vi "S_fi.vi"(6 "Parametry Ziemi":T1={"a - półoś duża"=6378137.0, "b - półoś mała"=6356752.3141999999998} {"b - półoś mała" format="%_20f"; "a - półoś duża" format="%_20g"}, 8 "E":ext, 9 "fi'":ext) -> (2 "S_fi":ext)   [LabVIEW 2015, in "Biblioteka moduł map v3.lvlib" / "Konwersja wsp.lvlib" / "UTM.lvlib" / "Konwersja z UTM na wsp geograficzne.lvlib"]
uses:
  Konwersja z UTM na wsp geograficzne.lvlib
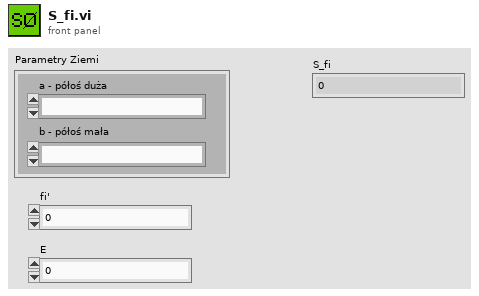
[diagram p1: front panel]
types:
  T1 = cluster{"a - półoś duża":ext, "b - półoś mała":ext}
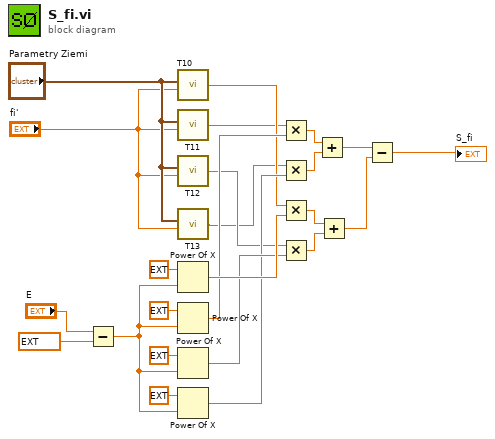
[diagram p0: block diagram]
diagram:
  n1 = Subtract(x="E", y=ext 500000.0 ("FE")) -> (x-y=w22:ext)
  n2 = call "T10.vi"("Parametry Ziemi"="Parametry Ziemi", "fi'"="fi'") -> ("T10"=w6:ext)  [unwired: 6 in]
  n3 = call "T11.vi"("Parametry Ziemi"="Parametry Ziemi", "fi'"="fi'") -> ("T11"=w5:ext)  [unwired: 6 in]
  n4 = call "T12.vi"("Parametry Ziemi"="Parametry Ziemi", "fi'"="fi'") -> ("T12"=w4:ext)  [unwired: 6 in]
  n5 = call "T13.vi"("Parametry Ziemi"="Parametry Ziemi", "fi'"="fi'") -> ("T13"=w3:ext)  [unwired: 6 in]
  n6 = Power Of X(1:w22, 2:ext 2.0 ("y")) -> (0:w17:ext)
  n7 = Power Of X(1:w22, 2:ext 4.0 ("y")) -> (0:w16:ext)
  n8 = Power Of X(1:w22, 2:ext 6.0 ("y")) -> (0:w15:ext)
  n9 = Power Of X(1:w22, 2:ext 8.0 ("y")) -> (0:w14:ext)
  n10 = Multiply(x=w5, y=w16) -> (x*y=w13:ext)
  n11 = Multiply(x=w3, y=w14) -> (x*y=w12:ext)
  n12 = Multiply(x=w6, y=w17) -> (x*y=w11:ext)
  n13 = Multiply(x=w4, y=w15) -> (x*y=w10:ext)
  n14 = Add(x=w13, y=w12) -> (x+y=w9:ext)
  n15 = Add(x=w11, y=w10) -> (x+y=w8:ext)
  n16 = Subtract(x=w9, y=w8) -> (x-y=→"S_fi":ext)
